vi "Encoder Example.vi"() -> ()   [LabVIEW 2012]
uses:
  <vilib>/LabVIEW Interface for Arduino/Type Defs/Board Type.ctl
  <vilib>/LabVIEW Interface for Arduino/LabVIEW Interface for Arduino.lvlib
panel:
  in  "Encoder Number":u8
  in  "stop":bool
  in  "Reset":bool
  out "Count":i32
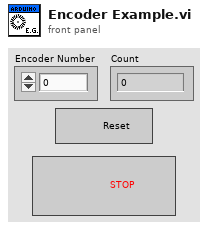
[diagram p1: front panel]
types:
  T1 = typedef "LabVIEW Interface for Arduino.lvlib/Board Type.ctl" = enum16{"Uno", "Dimuelanove w/Atmega 328", "Mega 2560"}
  T2 = typedef "LabVIEW Interface for Arduino.lvlib/Arduino Resource.ctl" = cluster{"VISA resource":refnum<visa-resource-name>, "Board Type":T1, "Connection Type":enum8{"USB / Serial"}, "Bytes Per Packet (15)":u8}
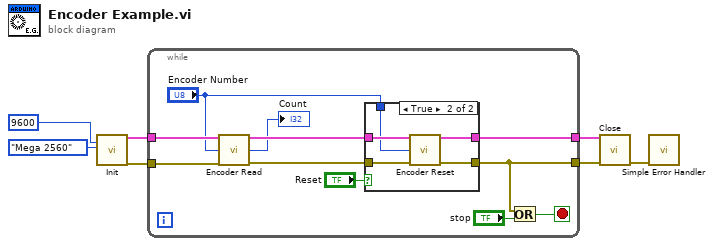
[diagram p0: block diagram]
diagram:
  n1 = call <vilib>:"Init.vi"("Baud Rate (115200)"=u32 9600, "Board Type (Uno)"=Board_Type."Mega 2560") -> ("Arduino Resource"=w7:T2, "error out"=w6:errorcluster)  [unwired: 16 in]
  n2 = while {
    tunnel: w7 -> [w18]
    tunnel: w6 -> [w14]
    tunnel: [w16] -> w5
    tunnel: [w9] -> w4
    stop <- w11 stop-if-true
    n3 = call "Encoder Read.vi"("Arduino Resource"=w18, "Encoder Number (0)"="Encoder Number", "error in"=w14) -> ("Arduino Resource Out"=w17:T2, "Count"=→"Count":i32, "error out"=w15:errorcluster)  [unwired: 10 in]
    n4 = case shown="True" "Reset" {
      tunnel: w17 -> [w20 w25]
      tunnel: [w20 w24] -> w16
      tunnel: [w19 w23] -> w9
      tunnel: w15 -> [w19 w22]
      tunnel: "Encoder Number" -> [_ w21]
      frame False {
      }
      frame True {
        n5 = call "Encoder Reset.vi"("Arduino Resource"=w25, "Encoder Number (0)"=w21, "error in"=w22) -> ("Arduino Resource Out"=w24:T2, "error out"=w23:errorcluster)  [unwired: 11 in]
      }
    }
    n6 = Or(x=w9, y="stop") -> (x .or. y?=w11:bool)
  }
  n7 = call <vilib>:"Close.vi"("Arduino Resource"=w5, "error in"=w4) -> ("error out"=w1:errorcluster)  [unwired: 13 in]
  n8 = call <vilib>:"Simple Error Handler.vi"("error in (no error)"=w1) -> ()  [unwired: 4 in, 5 out]
